vi "Set Legend.vi"(8 "error in (no error)":errorcluster, 9 "EMG?":bool=TRUE, 10 "Collection mode":T1=enum."Movement Input", 11 "Task Viewer in":refnum<class "Task Viewer.lvclass">) -> (0 "error out":errorcluster, 3 "Task Viewer out":refnum<class "Task Viewer.lvclass">)   [LabVIEW 2020, in "Task Viewer.lvlib" / "Task Viewer.lvclass"]
uses:
  Task Viewer.lvclass
  Collection Type df.ctl
  Task Viewer.lvclass/Task Viewer.ctl
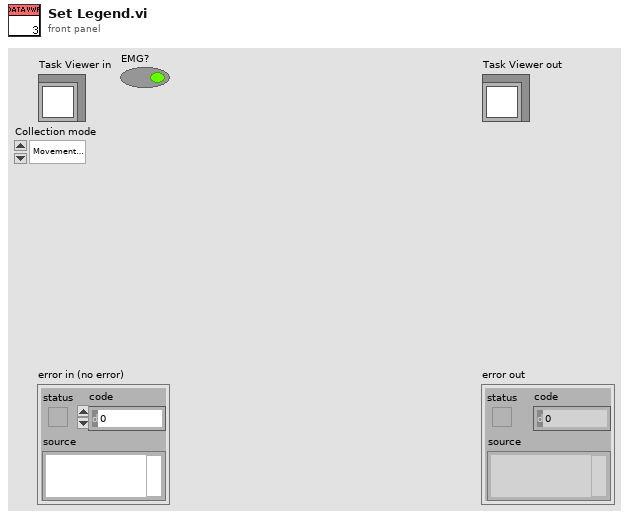
[diagram p1: front panel]
types:
  T1 = typedef "Collection Type df.ctl" = enum32{"Force Input", "Movement Input", "EMG only"}
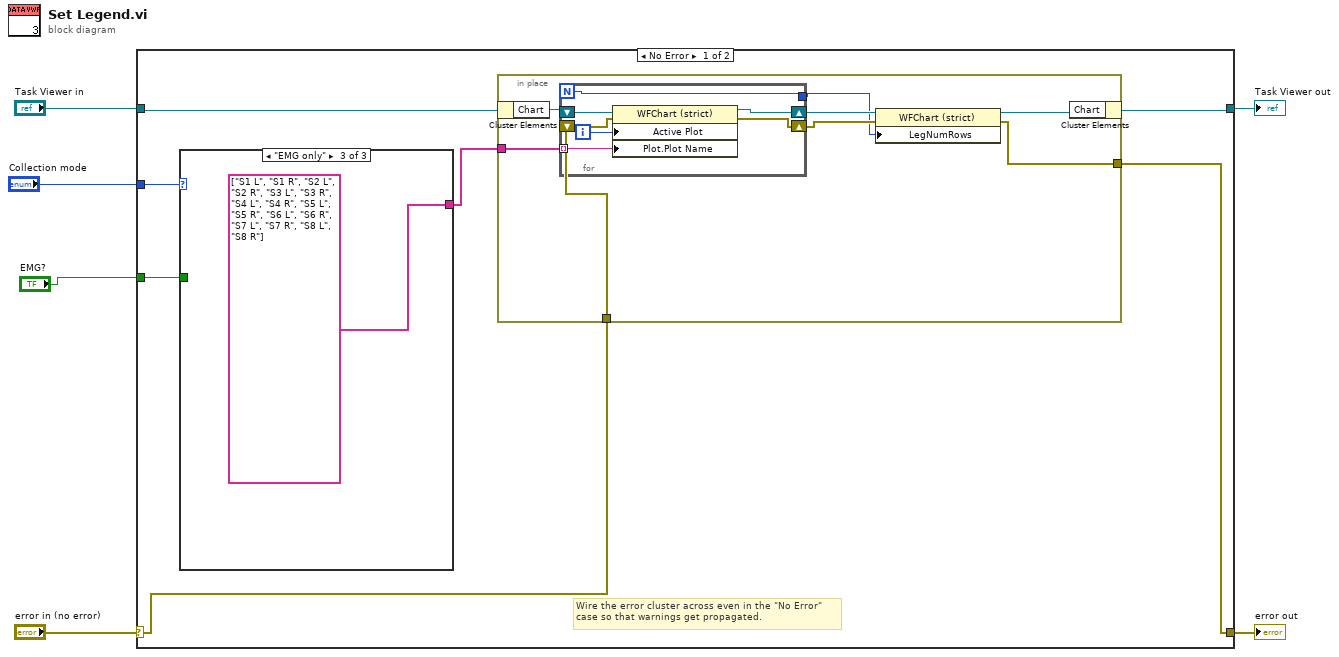
[diagram p0: block diagram]
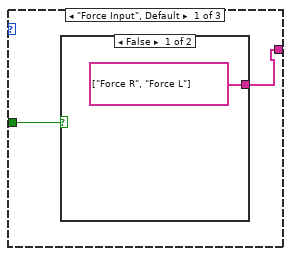
[diagram p2: hidden frame]
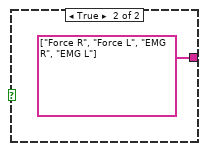
[diagram p3: hidden frame]
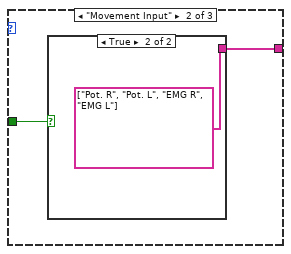
[diagram p4: hidden frame]
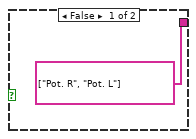
[diagram p5: hidden frame]
diagram:
  n1 = case shown="No Error" "error in (no error)" {
    selector: "error in (no error)" -> [w10 w38]
    tunnel: [w9 w38] -> w3
    tunnel: [w12 w39] -> w4
    tunnel: "Task Viewer in" -> [w13 w39]
    tunnel: "Collection mode" -> [w8 _]
    tunnel: "EMG?" -> [w7 _]
    frame No Error {
      # "Wire the error cluster across even in the \"No Error\"\ncase so that warnings get propagated."
      n2 = case shown="\"EMG only\"" w8 {
        tunnel: [w15 w19 string[] ["S1 L", "S1 R", "S2 L", "S2 R", "S3 L", "S3 R", "S4 L", "S4 R", "S5 L", "S5 R", "S6 L", "S6 R", "S7 L", "S7 R", "S8 L", "S8 R"]] -> w11
        tunnel: w7 -> [w14 w18 _]
        frame "Force Input", Default {
          n3 = case shown="False" w14 {
            tunnel: [string[] ["Force R", "Force L"] string[] ["Force R", "Force L", "EMG R", "EMG L"]] -> w15
            frame False {
            }
            frame True {
            }
          }
        }
        frame "Movement Input" {
          n4 = case shown="True" w18 {
            tunnel: [string[] ["Pot. R", "Pot. L"] string[] ["Pot. R", "Pot. L", "EMG R", "EMG L"]] -> w19
            frame False {
            }
            frame True {
            }
          }
        }
        frame "EMG only" {
        }
      }
      n5 = in-place {
        in-place-border: w11 -> [w29]
        in-place-border: w10 -> [w28]
        in-place-border: [w24] -> w9
        n6 = in-place-cluster #1(w13) -> ("Chart"=w30:refnum<vi>)
        n7 = for {
          N -> [w31]
          shift-right: [w36] -> w27
          shift-left: w30 -> [w37]
          tunnel: w29 -> [w34] mode=indexing
          shift-right: [w32] -> w25
          shift-left: w28 -> [w33]
          tunnel: [w31] -> w23
          i -> [w35]
          n8 = property class="WFChart (strict)"(reference=w37, error in=w33, "Active Plot"=w35, "Plot.Plot Name"=w34) -> (reference out=w36:refnum<vi>, error out=w32:errorcluster)
        }
        n9 = property class="WFChart (strict)"(reference=w27, error in=w25, "LegNumRows"=w23) -> (reference out=w26:refnum<vi>, error out=w24:errorcluster)
        n10 = in-place-cluster #1("Chart"=w26) -> (w12:refnum<class "Task Viewer.lvclass">)
      }
    }
    frame Error {
    }
  }
  "error out" <- w3
  "Task Viewer out" <- w4
